vi "Back_End_Chiller_PID.vi"(1 "Present Value":dbl=15.0 format="%.2f", 2 "Previous Control Sum":dbl format="%.2f", 3 "Setpoint":dbl=15.0 format="%.2f") -> (0 "Dem Output":dbl format="%.2f")   [LabVIEW 2010]
uses:
  <vilib>/Analysis/NI_AALPro.lvlib
panel:
  in  "O/P deadband":dbl=1.0 format="%.2f"
  in  "Kp Deadband":dbl format="%.2f"
  in  "Derivative History":i32=20
  out "deadbanded error":dbl format="%.2f"
  in  "P":bool=TRUE
  in  "D":bool=TRUE
  in  "I":bool=TRUE
  out "Waveform Chart":T1(graph)
  in  "Manual Demand":dbl min=0.0 max=100.0 format="%.2f"
  in  "Manual Override":bool
  out "Control Sum":dbl format="%.2f"
  out "Derivative Term":dbl format="%.2f"
  out "Integral Term":dbl format="%.2f"
  out "error differential":dbl format="%.5f"
  out "error integral":dbl format="%.2f"
  out "Proportional Term":dbl format="%.2f"
  in  "Kd":dbl=25.0 format="%.2f"
  in  "Ki":dbl=30.0 format="%.2f"
  in  "Kp":dbl=7.0 format="%.2f"
  out "error":dbl format="%.2f"
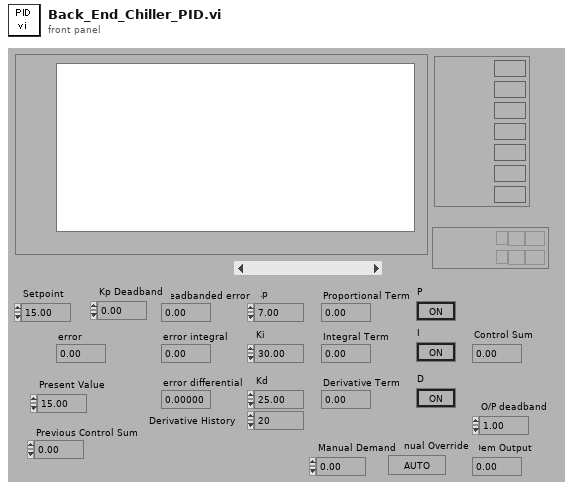
[diagram p1: front panel]
types:
  T1 = cluster{"Setpoint":dbl, "Present Value":dbl, "Proportional Term":dbl, "Integral Term":dbl, "Derivative Term":dbl, "Control Sum":dbl, "Dem Output":dbl}
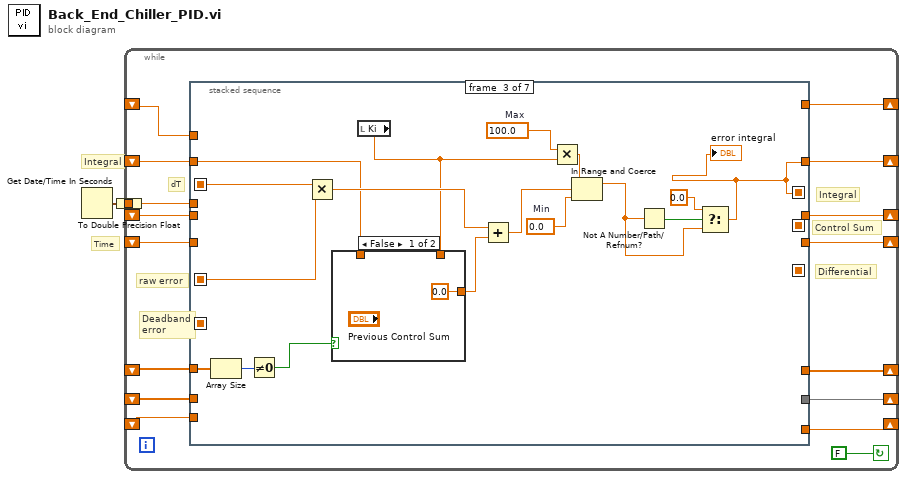
[diagram p0: block diagram]
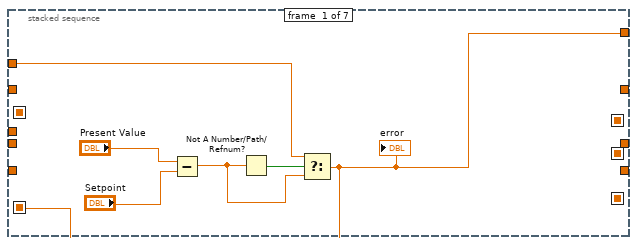
[diagram p2: hidden frame]
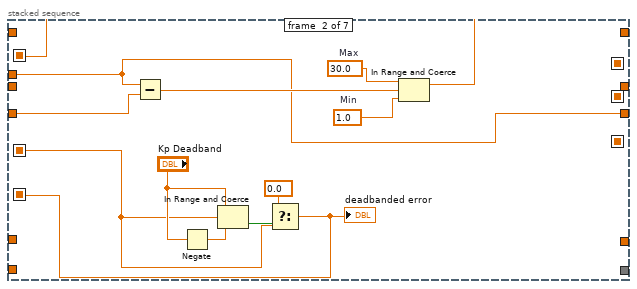
[diagram p3: hidden frame]
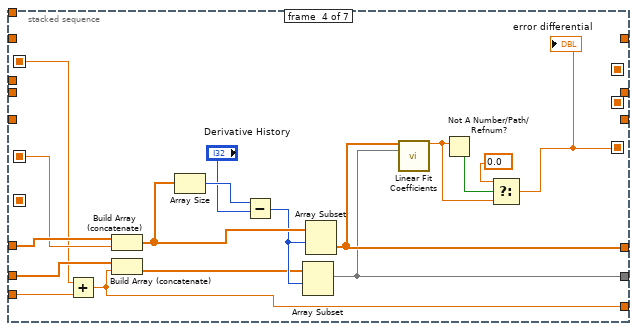
[diagram p5: hidden frame]
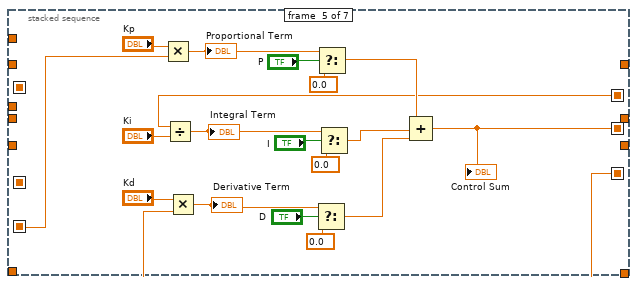
[diagram p6: hidden frame]
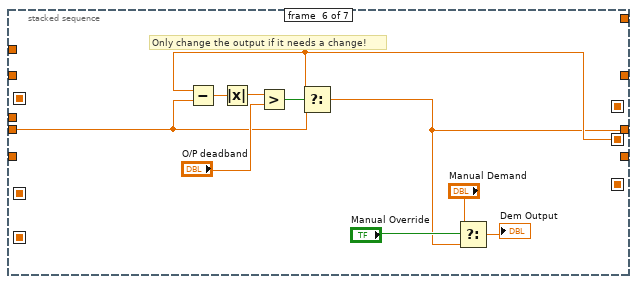
[diagram p7: hidden frame]
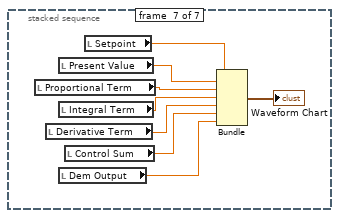
[diagram p8: hidden frame]
diagram:
  # "Integral"
  # "Time"
  n1 = Get Date/Time In Seconds() -> (seconds since 1Jan1904=w1:timestamp)
  n2 = To Double Precision Float(number=w1) -> (double precision float=w2:dbl)
  n3 = while {
    shift-left: _ -> [w5]
    shift-right: [w4] -> _
    shift-left: _ -> [w7]
    shift-right: [w6] -> _
    shift-left: _ -> [w9]
    shift-right: [w8] -> _
    tunnel: w2 -> [w14]
    shift-left: _ -> [w11]
    shift-right: [w10] -> _
    shift-left: _ -> [w13]
    shift-right: [w12] -> _
    shift-left: _ -> [w15]
    shift-right: [w16] -> _
    shift-left: _ -> [w18]
    shift-right: [w17] -> _
    stop <- FALSE continue-if-true
    # "Control Sum"
    # "raw error"
    # "Differential"
    # "Integral"
    # "Deadband\nerror"
    # "dT"
    n4 = stacked-sequence {
      seq-local: [_ w25 _ _ _ _ _] -> [_ _ w53 w58 _ _ _]
      seq-local: [_ w34 _ _ _ _ _] -> [_ _ _ _ w76 _ _]
      seq-local: [_ _ _ w63 _ _ _] -> [_ _ _ _ w75 _ _]
      seq-local: [_ _ w37 _ _ _ _] -> [_ _ _ _ w74 _ _]
      seq-local: [w19 _ _ _ _ _ _] -> [_ w26 w48 w64 _ _ _]
      seq-local: [_ _ _ _ w79 _ _] -> [_ _ _ _ _ w95 _]
      tunnel: w18 -> [_ w31 _ _ _ _ _]
      tunnel: [_ w29 _ _ _ _ _] -> w17
      tunnel: [_ _ w37 _ _ _ _] -> w16
      tunnel: w15 -> [_ _ w42 _ _ _ _]
      tunnel: w14 -> [_ w29 _ _ _ _ _]
      tunnel: w13 -> [_ _ w47 w72 _ _ _]
      tunnel: [_ _ _ w65 _ _ _] -> w12
      tunnel: w11 -> [_ _ _ w71 _ _ _]
      tunnel: [_ _ _ w62 _ _ _] -> w10
      tunnel: w9 -> [_ _ _ _ _ w93 _]
      tunnel: [_ _ _ _ _ w92 _] -> w8
      tunnel: w7 -> [_ _ _ w57 _ _ _]
      tunnel: [_ _ _ w56 _ _ _] -> w6
      tunnel: w5 -> [w21 _ _ _ _ _ _]
      tunnel: [w19 _ _ _ _ _ _] -> w4
      frame #0 {
        n5 = Subtract(x="Present Value", y="Setpoint") -> (x-y=w20:dbl)
        n6 = Not A Number/Path/Refnum?(number/path/refnum=w20) -> (NaN/Path/Refnum?=w22:bool)
        n7 = Select(t=w21, s=w22, f=w20) -> (s? t:f=w19:dbl)
        "error" <- w19
      }
      frame #1 {
        w32 = 1.0  # Min
        w33 = 30.0  # Max
        n8 = Subtract(x=w29, y=w31) -> (x-y=w30:dbl)
        n9 = Negate(x="Kp Deadband") -> (-x=w28:dbl)
        n10 = In Range and Coerce(upper limit="Kp Deadband", x=w26, lower limit=w28) -> (In Range?=w35:bool)  [unwired: 1 out]
        n11 = Select(t=0.0, s=w35, f=w26) -> (s? t:f=w34:dbl)
        "deadbanded error" <- w34
        n12 = In Range and Coerce(upper limit=w33, x=w30, lower limit=w32) -> (coerced(x)=w25:dbl)  [unwired: 1 out]
      }
      frame #2 {
        w52 = 0.0  # Min
        w51 = 100.0  # Max
        n13 = Array Size(array=w47) -> (size(s)=w46:i32)
        n14 = Not Equal To 0?(x=w46) -> (x != 0?=w44:bool)
        n15 = Multiply(x=w53, y=w48) -> (x*y=w45:dbl)
        n16 = local read "Ki"() -> (w41:dbl)
        n17 = case shown="False" w44 {
          tunnel: [0.0 ("Min") w55] -> w43
          tunnel: w42 -> [_ w55]
          tunnel: w41 -> [_ _]
          frame False {
          }
          frame True {
          }
        }
        n18 = Add(x=w45, y=w43) -> (x+y=w49:dbl)
        n19 = Multiply(x=w51, y=w41) -> (x*y=w50:dbl)
        n20 = In Range and Coerce(upper limit=w50, x=w49, lower limit=w52) -> (coerced(x)=w38:dbl)  [unwired: 1 out]
        n21 = Not A Number/Path/Refnum?(number/path/refnum=w38) -> (NaN/Path/Refnum?=w39:bool)
        n22 = Select(t=0.0, s=w39, f=w38) -> (s? t:f=w37:dbl)
        "error integral" <- w37
      }
      frame #3 {
        n23 = Add(x=w58, y=w57) -> (x+y=w56:dbl)
        n24 = Build Array (concatenate)(w72, w64) -> (w68:dbl[])
        n25 = Build Array (concatenate)(w71, w56) -> (w66:dbl[])
        n26 = Array Size(array=w68) -> (size(s)=w70:i32)
        n27 = Subtract(x=w70, y="Derivative History") -> (x-y=w67:i32)
        n28 = Array Subset(array=w66, index=w67) -> (w62:dbl[])  [unwired: 1 in]
        n29 = Array Subset(array=w68, index=w67) -> (w65:dbl[])  [unwired: 1 in]
        n30 = call <vilib>:"Linear Fit Coefficients.vi"("Y"=w65, "X"=w62) -> ("slope"=w59:dbl)  [unwired: 3 in, 10 out]
        n31 = Not A Number/Path/Refnum?(number/path/refnum=w59) -> (NaN/Path/Refnum?=w61:bool)
        n32 = Select(t=0.0 ("f"), s=w61, f=w59) -> (s? t:f=w63:dbl)
        "error differential" <- w63
      }
      frame #4 {
        n33 = Multiply(x="Kp", y=w76) -> (x*y=w89:dbl)
        "Proportional Term" <- w89
        n34 = Divide(x=w74, y="Ki") -> (x/y=w80:dbl)
        "Integral Term" <- w80
        n35 = Multiply(x="Kd", y=w75) -> (x*y=w81:dbl)
        "Derivative Term" <- w81
        n36 = Select(t=w81, s="D", f=0.0) -> (s? t:f=w83:dbl)
        n37 = Select(t=w89, s="P", f=0.0) -> (s? t:f=w90:dbl)
        n38 = Select(t=w80, s="I", f=0.0) -> (s? t:f=w82:dbl)
        n39 = Compound Arithmetic op=ADD(w90, w82, w83) -> (w79:dbl)
        "Control Sum" <- w79
      }
      frame #5 {
        # "Only change the output if it needs a change!"
        n40 = Subtract(x=w95, y=w93) -> (x-y=w98:dbl)
        n41 = Absolute Value(x=w98) -> (abs(x)=w97:dbl)
        n42 = Greater?(x=w97, y="O/P deadband") -> (0:w96:bool)
        n43 = Select(t=w95, s=w96, f=w93) -> (s? t:f=w92:dbl)
        n44 = Select(t="Manual Demand", s="Manual Override", f=w92) -> (s? t:f=→"Dem Output":dbl)
      }
      frame #6 {
        n45 = local read "Proportional Term"() -> (w105:dbl)
        n46 = local read "Derivative Term"() -> (w107:dbl)
        n47 = local read "Present Value"() -> (w104:dbl)
        n48 = local read "Integral Term"() -> (w106:dbl)
        n49 = local read "Dem Output"() -> (w109:dbl)
        n50 = local read "Control Sum"() -> (w108:dbl)
        n51 = local read "Setpoint"() -> (w103:dbl)
        n52 = Bundle("Setpoint"=w103, "Present Value"=w104, "Proportional Term"=w105, "Integral Term"=w106, "Derivative Term"=w107, "Control Sum"=w108, "Dem Output"=w109) -> (→"Waveform Chart":T1)  [unwired: 1 out]
      }
    }
  }
